vi "客户码.vi"(11 "追溯码":string) -> (3 "追溯码 2":string)   [LabVIEW 2020]
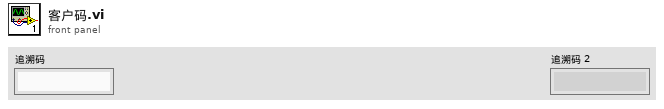
[diagram p1: front panel]
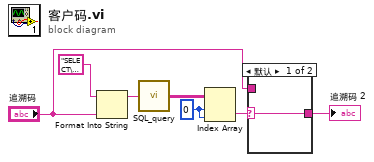
[diagram p0: block diagram]
diagram:
  w4 = 0 ("索引 (行)")
  n1 = Format Into String(format string="SELECT\ndbo.Code_Custom.CODE_MAIN\n\nFROM\ndbo.Code_Custom\nWHERE\ndbo.Code_Custom.CODE_CUSTOM = '%s'\n" ("格式字符串"), "追溯码") -> (resulting string=w6:string)  [unwired: 2 in, 1 out]
  n2 = call "SQL_query.vi"("SQL query"=w6) -> ("data"=w5:string[][])  [unwired: 3 in, 1 out]
  n3 = Index Array(array=w5, index (row)=w4, index (col)=w4) -> (element=w3:string)
  n4 = case shown="默认" w3 {
    selector: w3 -> [w8 _]
    tunnel: [w8 w9] -> w1
    tunnel: "追溯码" -> [_ w9]
    frame Default {
    }
    frame "" {
    }
  }
  "追溯码 2" <- w1
